vi "Right Side PWM.vi"(0 "Right rear":T1, 2 "Frequency":dbl format="%#_13g", 3 "Right Side Setpoint":dbl format="%.2f", 4 "Right Side Scale":dbl, 5 "Right PID Feedback":dbl format="%.2f", 6 "Right Mid":T1, 7 "Right Side Output Range":cluster{"output high":dbl, "output low":dbl}={"output high"=0.13333, "output low"=-0.13333} {"output low" format="%.5f"; "output high" format="%.5f"}, 8 "Right Front":T1, 9 "Right Side PID Gains":T8={"proportional gain (Kc)"=0.002, "integral time (Ti, min)"=7e-07, "derivative time (Td, min)"=0.0} {"derivative time (Td, min)" format="%.8f"; "integral time (Ti, min)" format="%.8f"; "proportional gain (Kc)" format="%.8f"}, 11 "Reset Right E.T.":bool caption="Reset") -> (15 "Right PWM":dbl, 17 "Right PID Output":dbl format="%.2f")   [LabVIEW 2015]
uses:
  <vilib>/myRIO/Instrument Drivers/Onboard IO/PWM/typedefs/PWM Reference.ctl
  <vilib>/myRIO/Common/Instrument Driver Framework/Utilities/typedefs/myRIO Generic Hardware Reference.ctl
  <vilib>/myRIO/Common/Instrument Driver Framework/Utilities/typedefs/Hardware Version Enum.ctl
  <vilib>/myRIO/Common/Instrument Driver Framework/Utilities/typedefs/myRIO v1.0 Reference.ctl
  <vilib>/myRIO/Common/Instrument Driver Framework/Utilities/typedefs/Generic FPGA Reference.ctl
  <vilib>/myRIO/Common/Instrument Driver Framework/myRIO v1.0/PWM/typedefs/PWM Channels Enum.ctl
  <vilib>/myRIO/Instrument Drivers/Onboard IO/PWM/typedefs/PWM Configuration.ctl
  <vilib>/addons/control/pid/pid.llb/PID (DBL).vi
  <vilib>/Utility/error.llb/Error Cluster From Error Code.vi
  <vilib>/myRIO/Common/Instrument Driver Framework/myRIO v1.0/PWM/vis/myRIO v1.0 Write PWM.vi
  <vilib>/myRIO/Instrument Drivers/Onboard IO/PWM/PWM.lvlib
  <vilib>/addons/control/pid/NI_PID_pid.lvlib
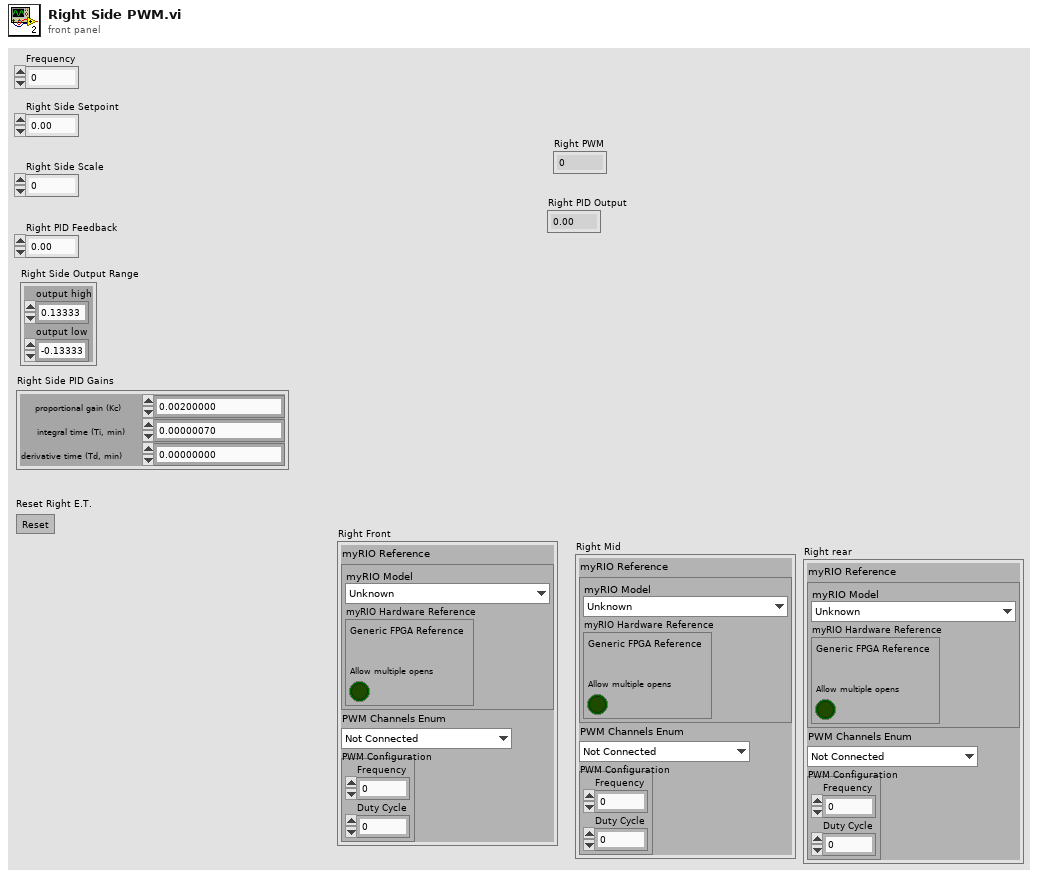
[diagram p1: front panel]
types:
  T1 = typedef "PWM.lvlib/PWM Reference.ctl" = cluster{"myRIO Reference":T2, "PWM Channels Enum":T6, "PWM Configuration":T7}
  T2 = typedef "myRIO Generic Hardware Reference.ctl" = cluster{"myRIO Model":T3, "myRIO Hardware Reference":T4}
  T3 = typedef "Hardware Version Enum.ctl" = enum16{"Unknown", "myRIO-1900", "myRIO-1950", "roboRIO"}
  T4 = typedef "myRIO v1.0 Reference.ctl" = cluster{"Generic FPGA Reference":T5, "Allow multiple opens":bool}
  T5 = typedef "Generic FPGA Reference.ctl" = refnum<k20>
  T6 = typedef "PWM Channels Enum.ctl" = enum16{"Not Connected", "C/PWM0", "C/PWM1", "A/PWM0", "A/PWM1", "A/PWM2", "B/PWM0", "B/PWM1", "B/PWM2", "PWM/PWM0", "PWM/PWM1", "PWM/PWM2", "PWM/PWM3", "PWM/PWM4", "PWM/PWM5", "PWM/PWM6", "PWM/PWM7", "PWM/PWM8", "PWM/PWM9"}
  T7 = typedef "PWM.lvlib/PWM Configuration.ctl" = cluster{"Frequency":dbl, "Duty Cycle":dbl}
  T8 = cluster{"proportional gain (Kc)":dbl, "integral time (Ti, min)":dbl, "derivative time (Td, min)":dbl}
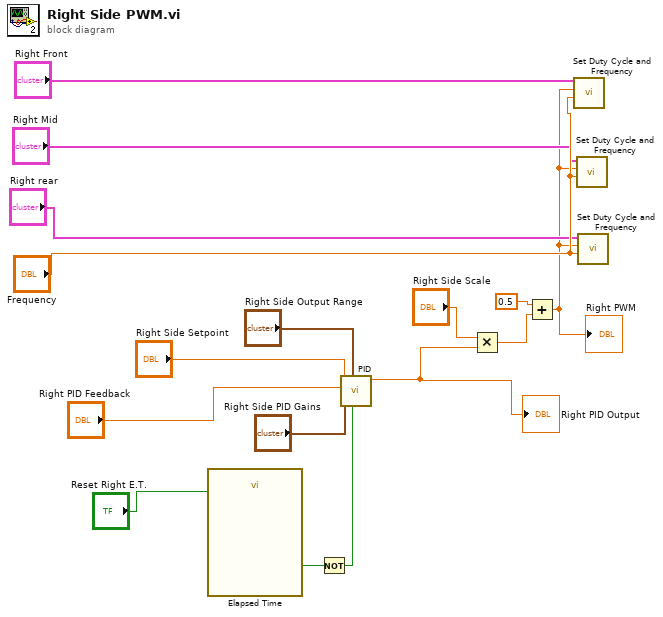
[diagram p0: block diagram]
diagram:
  n1 = call "Elapsed Time"("Reset"="Reset Right E.T.") -> ("Time has Elapsed"=w4:bool)  [unwired: 11 in, 7 out]
  n2 = Not(x=w4) -> (.not. x?=w3:bool)
  n3 = call-poly <vilib>:"PID.vi"("reinitialize? (F)"=w3, "output range"="Right Side Output Range", "PID gains"="Right Side PID Gains", "process variable"="Right PID Feedback", "setpoint"="Right Side Setpoint") -> ("output"=w9:dbl)  [unwired: 5 in, 1 out]
  "Right PID Output" <- w9
  n4 = Multiply(x="Right Side Scale", y=w9) -> (x*y=w7:dbl)
  n5 = Add(x=0.5, y=w7) -> (x+y=w5:dbl)
  "Right PWM" <- w5
  n6 = call <vilib>:"Set Duty Cycle and Frequency.vi"("Frequency [Hz]"="Frequency", "Duty Cycle"=w5, "PWM Ref In"="Right Front") -> ()  [unwired: 6 in, 2 out]
  n7 = call <vilib>:"Set Duty Cycle and Frequency.vi"("Frequency [Hz]"="Frequency", "Duty Cycle"=w5, "PWM Ref In"="Right Mid") -> ()  [unwired: 6 in, 2 out]
  n8 = call <vilib>:"Set Duty Cycle and Frequency.vi"("Frequency [Hz]"="Frequency", "Duty Cycle"=w5, "PWM Ref In"="Right rear") -> ()  [unwired: 6 in, 2 out]
